vi "System@Log Error__Parameter.vi"(1 "ParamterIn":string) -> (0 "ParamterOut":string)   [LabVIEW 2019]
panel:
  in  "Message":string(combo)
  in  "Confirm":bool
  # "System@Log Error $Error Message"
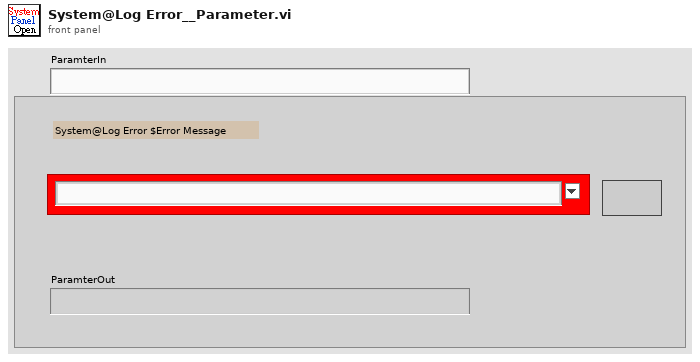
[diagram p1: front panel]
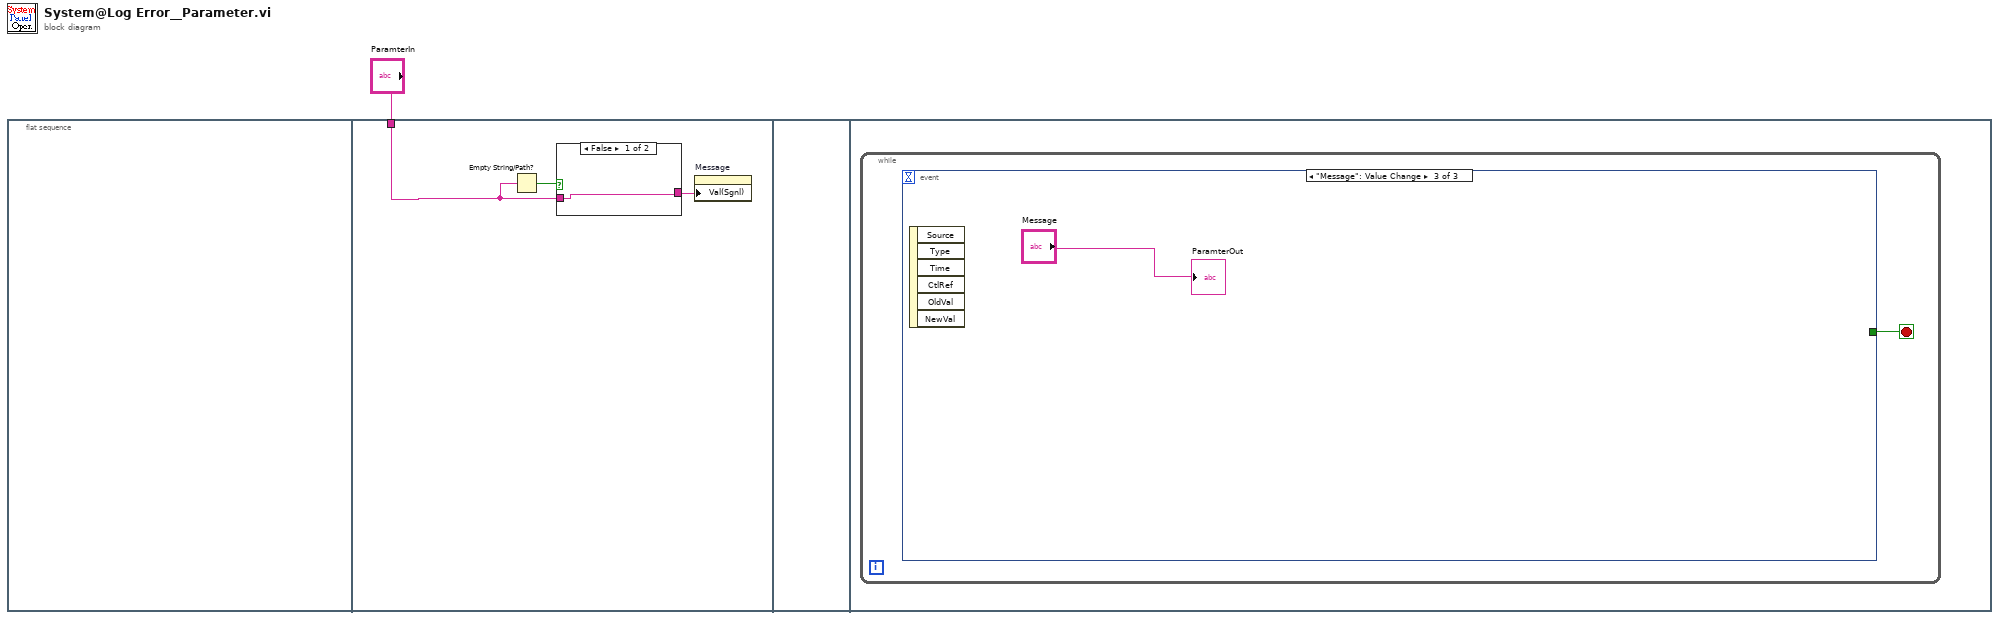
[diagram p0: block diagram]
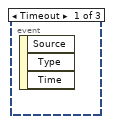
[diagram p3: hidden frame]
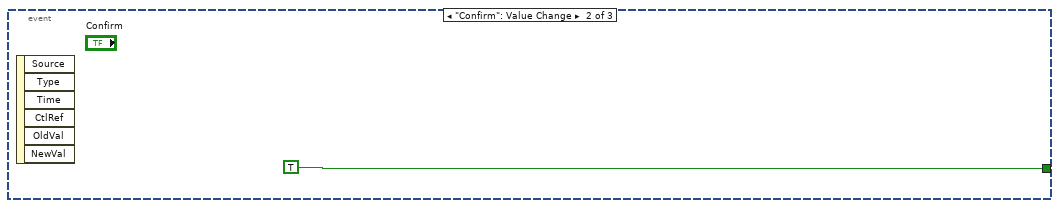
[diagram p4: hidden frame]
diagram:
  n1 = flat-sequence {
    tunnel: "ParamterIn" -> [w2]
    frame #0 {
    }
    frame #1 {
      n2 = Empty String/Path?(string/path=w2) -> (empty?=w4:bool)
      n3 = case shown="False" w4 {
        tunnel: w2 -> [w5 w6]
        tunnel: [w5 w6] -> w3
        frame False {
        }
        frame True {
        }
      }
      n4 = property on="Message" class="CmbBox"("Val(Sgnl)"=w3) -> ()  [unwired: 2 in, 2 out]
    }
    frame #2 {
    }
    frame #3 {
      n5 = while {
        stop <- w7 stop-if-true
        n6 = event shown="[2] \"Message\": Value Change" {
          selector: _ -> [_ _ _]
          dyn-events: _ -> [_ _ _]
          timeout: _ -> [_ _ _]
          tunnel: [_ TRUE _] -> w7
          event Timeout {
            n7 = event-data() -> ()  [unwired: 1 in, 3 out]
          }
          event "Confirm": Value Change {
            n8 = event-data() -> ()  [unwired: 1 in, 6 out]
          }
          event "Message": Value Change {
            n9 = event-data() -> ()  [unwired: 1 in, 6 out]
            "ParamterOut" <- "Message"
          }
        }
      }
    }
  }
